vi "Initialize Match Template.vi"(11 "base path":path=path "Fiducial_3_Dots.bmp") -> (3 "Pattern Matched Image":T1(plugin-control))   [LabVIEW 2018]
uses:
  <vilib>/vision/NI_Vision_Development_Module.lvlib
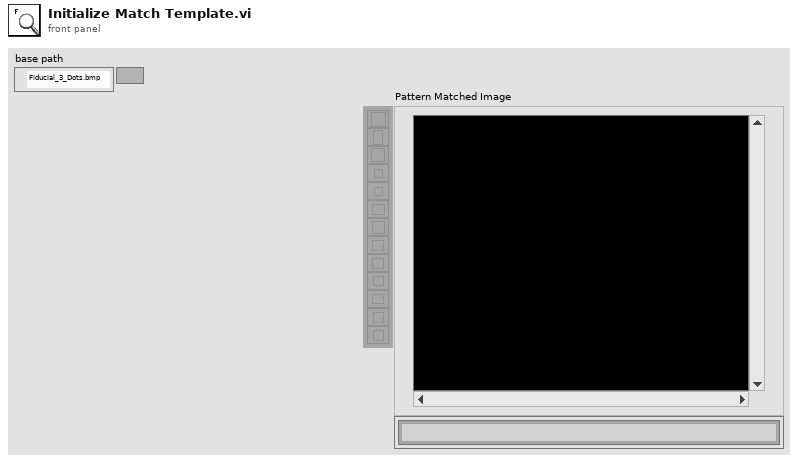
[diagram p1: front panel]
types:
  T1 = typedef "IMAQ Image.ctl" = refnum<image>
  T2 = typedef "Image Type" = u32
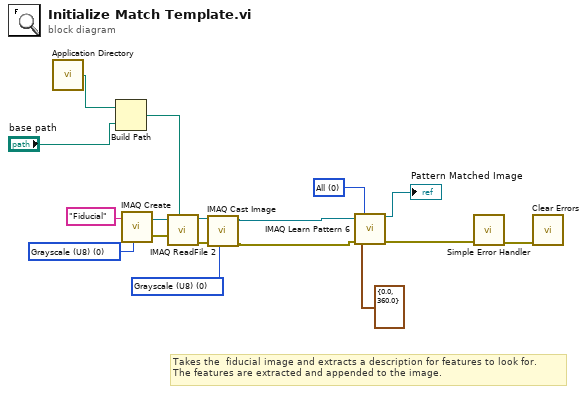
[diagram p0: block diagram]
diagram:
  w6 = T2 0 items=["Grayscale (U8)", "Grayscale (I16)", "Grayscale (SGL)", "Complex (CSG)", "RGB (U32)", "HSL (U32)", "RGB (U64)", "Grayscale (U16)"] ("Image Type")
  w10 = T2 0 items=["Grayscale (U8)", "Grayscale (I16)", "Grayscale (SGL)", "Complex (CSG)", "RGB (U32)", "HSL (U32)", "RGB (U64)", "Grayscale (U16)"] ("Image Type")
  w14 = 0 items=["All", "Low Discrepancy Sampling", "Grayscale Value Pyramid", "Gradients Pyramid"] ("Algorithm")
  # "Takes the  fiducial image and extracts a description for features to look for.\nThe features are extracted and appended to the image."
  n1 = call <vilib>:"Application Directory.vi"() -> ("Application Directory"=w3:path)
  n2 = Build Path(base path=w3, name or relative path="base path") -> (appended path=w1:path)
  n3 = call "IMAQ Create"("Image Name"="Fiducial", "Image Type"=w10) -> ("New Image"=w9:T1, "error out"=w12:errorcluster)  [unwired: 3 in]
  n4 = call "IMAQ ReadFile 2"("File Path"=w1, "error in (no error)"=w12, "Image"=w9) -> ("error out"=w8:errorcluster, "Image Out"=w7:T1)  [unwired: 4 in, 3 out]
  n5 = call "IMAQ Cast Image"("Image Type"=w6, "error in (no error)"=w8, "Image Src"=w7) -> ("error out"=w5:errorcluster, "Image Dst Out"=w4:T1)  [unwired: 7 in]
  n6 = call "IMAQ Learn Pattern 6"("Image"=w4, "Algorithm"=w14, "Angle Range"=cluster{"Start Angle":sgl, "End Angle":sgl} {"Start Angle"=0.0, "End Angle"=360.0}, "error in (no error)"=w5) -> ("Template Image Out"=→"Pattern Matched Image":T1, "error out"=w16:errorcluster)  [unwired: 9 in, 1 out]
  n7 = call <vilib>:"Simple Error Handler.vi"("error in (no error)"=w16) -> ("error out"=w17:errorcluster)  [unwired: 4 in, 4 out]
  n8 = call <vilib>:"Clear Errors.vi"("error in (no error)"=w17) -> ()  [unwired: 5 in, 2 out]
